vi "RTsave Thread.vi"   [LabVIEW 2011, in "CAN FD.lvlib"]
uses:
  CAN FD.lvlib
  Typedef/CAN Data.ctl
types:
  T1 = enum16{"deny read/write", "deny write-only", "deny none"}
  T2 = enum16{"open", "replace", "create", "open or create", "replace or create", "replace or create with confirmation"}
  T3 = typedef "CAN FD.lvlib/CAN Data.ctl" = cluster{"SystemTime":timestamp, "HwTime":dbl, "Channel":u8, "ID":u32, "CANType":i16, "Direction":i16, "Remote":bool, "Ext":bool, "Len":u8, "Data":u8[], "Success":bool}
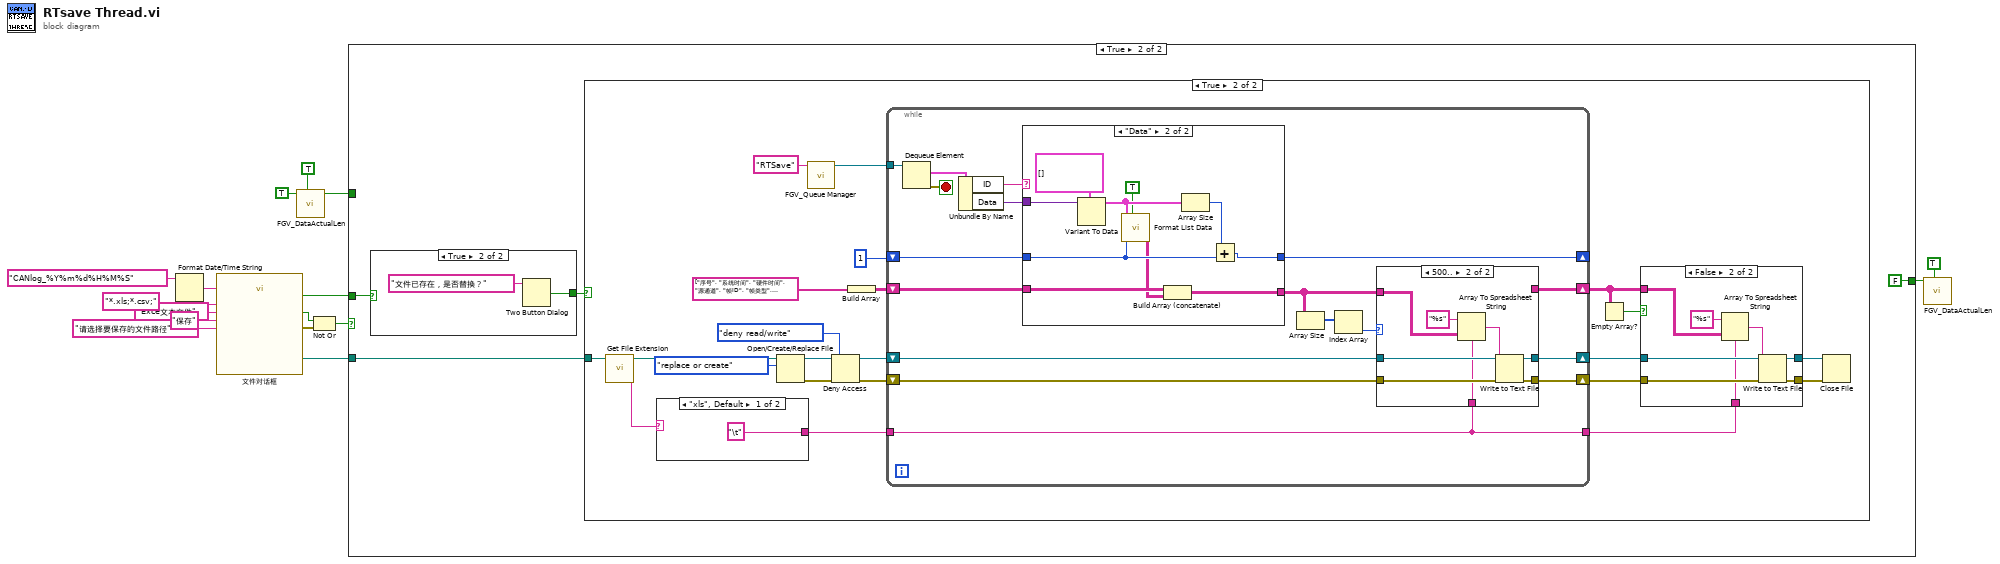
[diagram p0: block diagram]
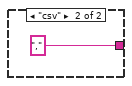
[diagram p5: hidden frame]
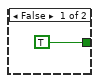
[diagram p8: hidden frame]
diagram:
  w1 = "保存" ("button label")
  (unwired) "Exce文本文件" ("pattern (all files)")
  n1 = Format Date/Time String(time format string (%c)="CANlog_%Y%m%d%H%M%S" ("时间格式字符串(%c)")) -> (date/time string=w14:string)  [unwired: 2 in]
  n2 = call "文件对话框"("prompt"="请选择要保存的文件路径", "button label"=w1, "default name"=w14, "pattern (all files)"="*.xls;*.csv;" ("pattern label"), "pattern label"=w1) -> ("selected path"=w9:path, "exists"=w8:bool, "cancelled"=w11:bool, "error out"=w12:errorcluster)  [unwired: 7 in]
  n3 = call "FGV_DataActualLen.vi"("Set"=TRUE, "RTsave"=TRUE) -> ("RTsave"=w5:bool)  [unwired: 8 in, 1 out]
  n4 = Not Or(1:w12, 2:w11) -> (0:w10:bool)
  n5 = case shown="True" w10 {
    tunnel: w9 -> [_ w17]
    tunnel: w8 -> [_ w19]
    tunnel: w5 -> [_ _]
    tunnel: [_ FALSE] -> w4
    frame False {
    }
    frame True {
      n6 = case shown="True" w19 {
        tunnel: [TRUE ("T button?") w95] -> w18
        frame False {
        }
        frame True {
          n7 = Two Button Dialog(message="文件已存在，是否替换？" ("消息")) -> (T button?=w95:bool)  [unwired: 2 in]
        }
      }
      n8 = case shown="True" w18 {
        tunnel: w17 -> [_ w31]
        frame False {
        }
        frame True {
          n9 = call <vilib>:"Get File Extension.vi"("file"=w31) -> ("lowercase file extension"=w29:string, "dup file"=w30:path)  [unwired: 7 in, 2 out]
          n10 = case shown="\"xls\", Default" w29 {
            tunnel: ["\t" ","] -> w28
            frame "xls", Default {
            }
            frame "csv" {
            }
          }
          n11 = Open/Create/Replace File(file path (use dialog)=w30, operation (0:open)=T2."replace or create" ("操作(0:open)")) -> (refnum out=w39:refnum<file>, error out=w38:errorcluster)  [unwired: 4 in, 1 out]
          n12 = call "FGV_Queue Manager.vi"("Name"="RTSave") -> ("Queue"=w33:refnum<queue>)  [unwired: 8 in, 2 out]
          n13 = Deny Access(4:w38, 6:T1."deny read/write" ("限制模式(0:读/写限制)"), 7:w39) -> (0:w37:errorcluster, 3:w36:refnum<file>)
          n14 = Build Array(string[] ["序号", "系统时间", "硬件时间", "源通道", "帧ID", "帧类型", "帧格式", "CAN类型", "方向", "长度", "数据"]) -> (w34:string[][])
          n15 = while {
            shift-right: [w56] -> w25
            shift-left: w34 -> [w62]
            tunnel: w33 -> [w66]
            shift-right: [w60] -> _
            shift-left: 1 -> [w61]
            tunnel: w28 -> [w54]
            shift-right: [w69] -> w24
            shift-left: w36 -> [w67]
            shift-right: [w70] -> w23
            shift-left: w37 -> [w68]
            tunnel: [w54] -> w20
            stop <- w55 stop-if-true
            n16 = Dequeue Element(queue=w66) -> (element=w65:cluster{"ID":string, "Data":variant}, error out=w55:errorcluster)  [unwired: 2 in, 2 out]
            n17 = Unbundle By Name(w65) -> ("ID"=w64:string, "Data"=w63:variant)
            n18 = case shown="\"Data\"" w64 {
              tunnel: w63 -> [_ w93]
              tunnel: w62 -> [w82 w87]
              tunnel: w61 -> [w83 w90]
              tunnel: [w83 w88] -> w60
              tunnel: [w82 w85] -> w57
              frame Default {
              }
              frame "Data" {
                n19 = Variant To Data(type=T3[] [], Variant=w93) -> (data=w91:T3[])  [unwired: 1 in, 1 out]
                n20 = call "Format List Data.vi"("Include All time"=TRUE, "#Offset"=w90, "Data"=w91) -> ("List Data"=w86:string[][])  [unwired: 8 in]
                n21 = Build Array (concatenate)(w87, w86) -> (w85:string[][])
                n22 = Array Size(array=w91) -> (size(s)=w89:i32)
                n23 = Add(x=w89, y=w90) -> (x+y=w88:i32)
              }
            }
            n24 = Array Size(array=w57) -> (size(s)=w59:i32[])
            n25 = Index Array(array=w59) -> (element=w58:i32)  [unwired: 1 in]
            n26 = case shown="500.." w58 {
              tunnel: [w72 w79] -> w70
              tunnel: [w73 w78] -> w69
              tunnel: w68 -> [w72 w77]
              tunnel: w67 -> [w73 w76]
              tunnel: w57 -> [w71 w75]
              tunnel: [w71 _] -> w56
              tunnel: w54 -> [_ w74]
              frame 0, Default {
              }
              frame 500.. {
                n27 = Array To Spreadsheet String(delimiter (Tab)=w74, array=w75, 3:"%s" ("格式字符串")) -> (spreadsheet string=w80:string)
                n28 = Write to Text File(file (use dialog)=w76, text=w80, error in=w77) -> (refnum out=w78:refnum<file>, error out=w79:errorcluster)  [unwired: 1 in, 1 out]
              }
            }
          }
          n29 = Empty Array?(array=w25) -> (empty?=w26:bool)
          n30 = case shown="False" w26 {
            tunnel: [w42 w49] -> w21
            tunnel: [w43 w48] -> w22
            tunnel: w23 -> [w42 w47]
            tunnel: w24 -> [w43 w46]
            tunnel: w25 -> [_ w45]
            tunnel: w20 -> [_ w44]
            frame True {
            }
            frame False {
              n31 = Array To Spreadsheet String(delimiter (Tab)=w44, array=w45, 3:"%s" ("格式字符串")) -> (spreadsheet string=w50:string)
              n32 = Write to Text File(file (use dialog)=w46, text=w50, error in=w47) -> (refnum out=w48:refnum<file>, error out=w49:errorcluster)  [unwired: 1 in, 1 out]
            }
          }
          n33 = Close File(refnum=w22, error in=w21) -> ()  [unwired: 2 out]
        }
      }
    }
  }
  n34 = call "FGV_DataActualLen.vi"("Set"=TRUE, "RTsave"=w4) -> ()  [unwired: 8 in, 2 out]
